vi "Test Message.vi"(8 "error in (no error)":errorcluster) -> (0 "error out":errorcluster)   [LabVIEW 2020]
uses:
  Source/Protobuf RAW/double/double.lvclass/double.ctl
  Source/Protobuf RAW/sint64/sint64.lvclass/sint64.ctl
  Source/Protobuf RAW/string/string.lvclass/string.ctl
  Source/Protobuf RAW/int32/int32.lvclass/int32.ctl
  Source/Protobuf RAW/sint64/Write Value.vi
  Source/Protobuf RAW/double/Write Value.vi
  Source/Protobuf RAW/string/Write Value.vi
  Source/Protobuf RAW/int32/Write Value.vi
  Source/Protobuf RAW/string/string.lvclass
  E:/Labview/LV 2020/Libs/LV Protobuf Raw/Source/Protobuf RAW/Tag/Basic Type.lvclass
  Source/Protobuf RAW/double/double.lvclass
  Source/Protobuf RAW/sint64/sint64.lvclass
  Source/Protobuf RAW/int32/int32.lvclass
  Source/Protobuf RAW/Message/New Raw Message.vi
  <vilib>/addons/_JKI Toolkits/Caraya/classes/Assert/Assert Equal Value_Variant.vi
  <vilib>/addons/_JKI Toolkits/Caraya/classes/Assert/Assert Not Equal Value_Variant.vi
  Source/Protobuf RAW/Message/Raw Message.lvclass
  Source/Protobuf RAW/Tag/Basic Type.lvclass
  <vilib>/addons/_JKI Toolkits/Caraya/classes/Test/Test.lvclass
  Source/Protobuf RAW.lvlib
  <vilib>/addons/_JKI Toolkits/Caraya/classes/Assert/Assert.lvclass
  E:/Labview/LV 2020/Libs/LV Protobuf Raw/Source/Protobuf RAW/Proto Value/Proto Type.lvclass
  E:/Labview/LV 2020/Libs/LV Protobuf Raw/Source/Protobuf RAW/Type Serializer/Type Serializer.lvclass
  E:/Labview/LV 2020/Libs/LV Protobuf Raw/Source/Protobuf RAW/String Representable/String Representable.lvclass
  E:/Labview/LV 2020/Libs/LV Protobuf Raw/Source/Protobuf RAW/Wire Type Group/Wire Type Group.lvclass
  E:/Labview/LV 2020/Libs/LV Protobuf Raw/Source/Protobuf RAW/LEN Encoder/LEN.lvclass
  E:/Labview/LV 2020/Libs/LV Protobuf Raw/Source/Protobuf RAW/string/string.lvclass
  E:/Labview/LV 2020/Libs/LV Protobuf Raw/Source/Protobuf RAW/Scalar Encoder/Scalar Type.lvclass
  E:/Labview/LV 2020/Libs/LV Protobuf Raw/Source/Protobuf RAW/VarINT Encoder/VarINT.lvclass
  E:/Labview/LV 2020/Libs/LV Protobuf Raw/Source/Protobuf RAW/int32/int32.lvclass
  E:/Labview/LV 2020/Libs/LV Protobuf Raw/Source/Protobuf RAW/I64 Wire/I64.lvclass
  E:/Labview/LV 2020/Libs/LV Protobuf Raw/Source/Protobuf RAW/double/double.lvclass
  E:/Labview/LV 2020/Libs/LV Protobuf Raw/Source/Protobuf RAW/Message/Raw Message.lvclass
  E:/Labview/LV 2020/Libs/LV Protobuf Raw/Source/Protobuf RAW/sint64/sint64.lvclass
panel:
  out "String Representation":string
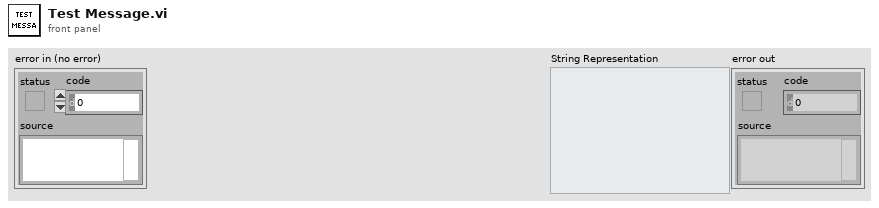
[diagram p1: front panel]
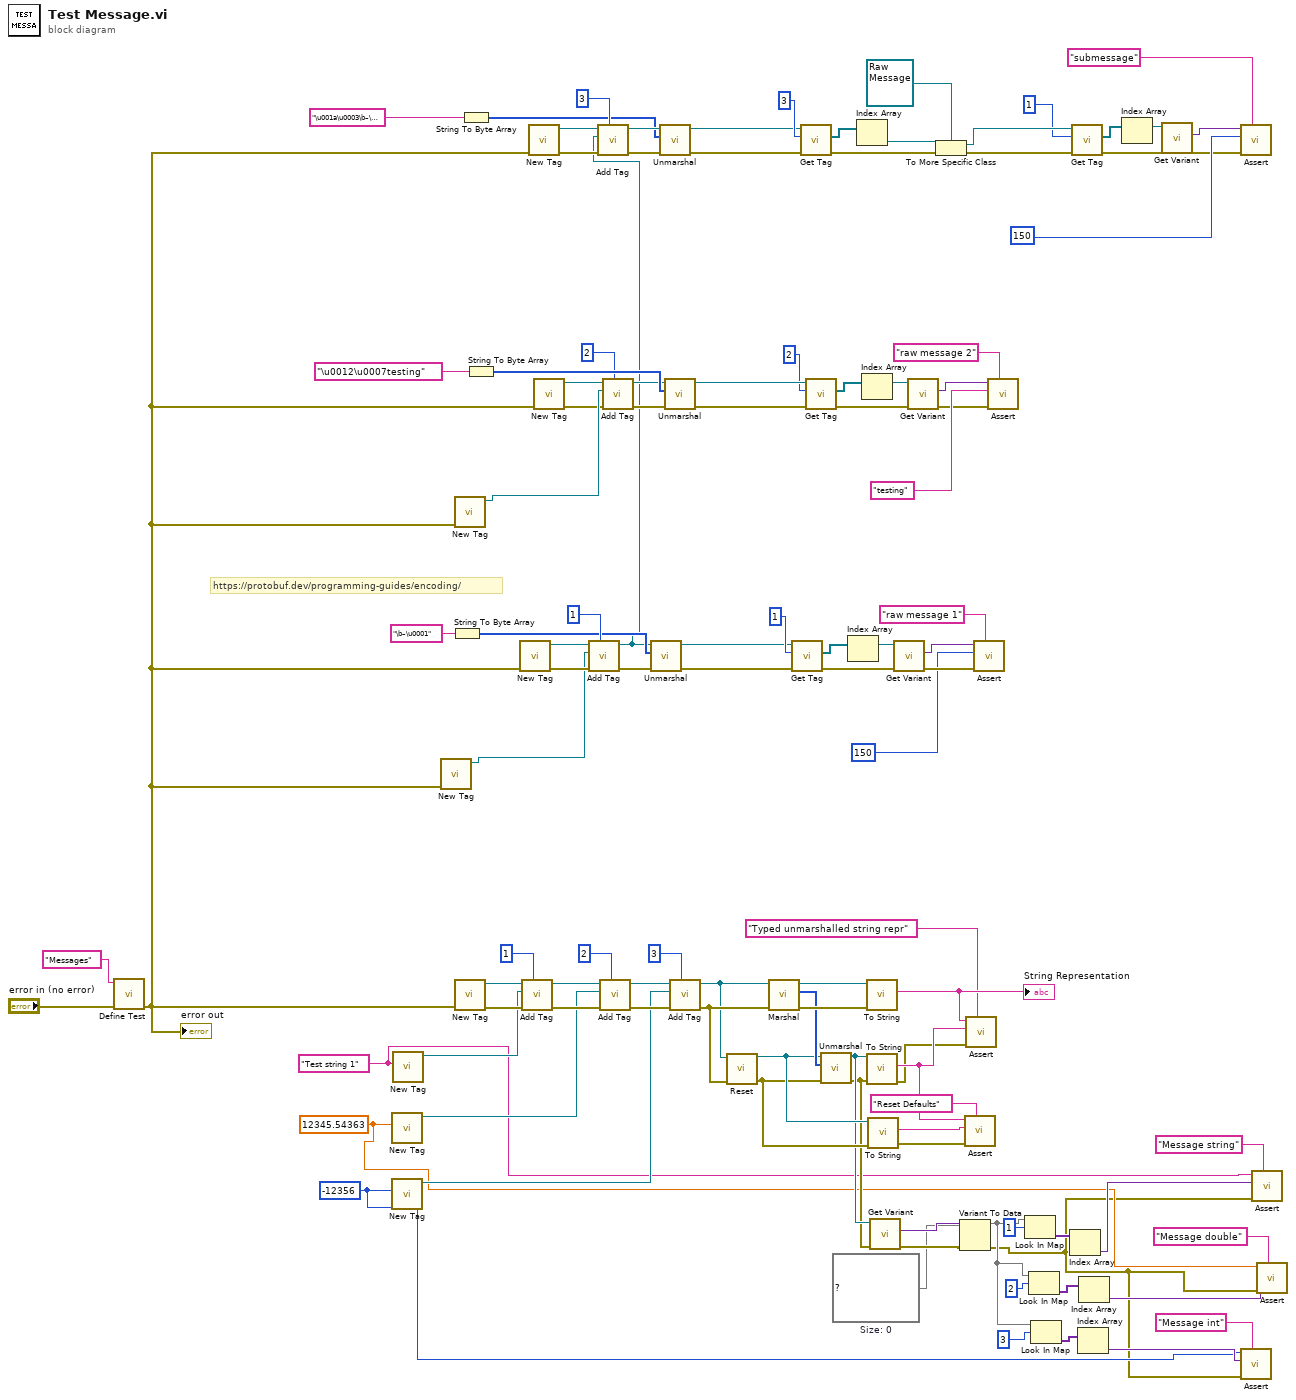
[diagram p0: block diagram]
diagram:
  w81 = map{u32, variant[]} {}  # Size: 0
  w69 = i64 -12356 ("Value")
  w68 = 12345.54363 ("Value")
  w73 = "Test string 1" ("Value")
  # "https://protobuf.dev/programming-guides/encoding/"
  n1 = call <vilib>:"Define Test.vi"("error in (no error)"="error in (no error)", "Label (VI Title)"="Messages") -> ("error out"=w12:errorcluster)  [unwired: 9 in]
  "error out" <- w12
  n2 = call-poly "New Tag.vi"("Value"=w68) -> ("double out"=w102:refnum<class "double.lvclass">)  [unwired: 9 in, 1 out]
  n3 = call-poly "New Tag.vi"("Value"=w69) -> ("int32 out"=w98:refnum<class "sint64.lvclass">)  [unwired: 9 in, 1 out]
  n4 = call-poly "New Tag.vi"("Value"=w73) -> ("string out"=w106:refnum<class "string.lvclass">)  [unwired: 9 in, 1 out]
  n5 = call-poly "New Tag.vi"("error in (no error)"=w12) -> ("int32 out"=w59:refnum<class "int32.lvclass">)  [unwired: 9 in, 1 out]
  n6 = String To Byte Array(string="\b–\u0001") -> (unsigned byte array=w48:u8[])
  n7 = call-poly "New Tag.vi"("error in (no error)"=w12) -> ("string out"=w30:refnum<class "string.lvclass">)  [unwired: 9 in, 1 out]
  n8 = call-poly "New Tag.vi"("error in (no error)"=w12) -> ("error out"=w108:errorcluster, "Raw Message out"=w109:refnum<class "Raw Message.lvclass">)  [unwired: 9 in]
  n9 = String To Byte Array(string="\u001a\u0003\b–\u0001") -> (unsigned byte array=w16:u8[])
  n10 = String To Byte Array(string="\u0012\u0007testing") -> (unsigned byte array=w41:u8[])
  n11 = call-poly "New Tag.vi"("error in (no error)"=w12) -> ("error out"=w60:errorcluster, "Raw Message out"=w61:refnum<class "Raw Message.lvclass">)  [unwired: 9 in]
  n12 = call-dynamic "Add Tag.vi"("ID"=u32 1, "error in (no error)"=w108, "Tag Value"=w106, "Message in"=w109) -> ("error out"=w105:errorcluster, "Message out"=w104:refnum<class "Raw Message.lvclass">)  [unwired: 6 in]
  n13 = call-poly "New Tag.vi"("error in (no error)"=w12) -> ("error out"=w24:errorcluster, "Raw Message out"=w25:refnum<class "Raw Message.lvclass">)  [unwired: 9 in]
  n14 = call-poly "New Tag.vi"("error in (no error)"=w12) -> ("error out"=w29:errorcluster, "Raw Message out"=w28:refnum<class "Raw Message.lvclass">)  [unwired: 9 in]
  n15 = call-dynamic "Add Tag.vi"("ID"=u32 1, "error in (no error)"=w60, "Tag Value"=w59, "Message in"=w61) -> ("error out"=w58:errorcluster, "Message out"=w13:refnum<class "Raw Message.lvclass">)  [unwired: 6 in]
  n16 = call-dynamic "Add Tag.vi"("ID"=u32 3, "error in (no error)"=w24, "Tag Value"=w13, "Message in"=w25) -> ("error out"=w23:errorcluster, "Message out"=w22:refnum<class "Raw Message.lvclass">)  [unwired: 6 in]
  n17 = call-dynamic "Add Tag.vi"("ID"=u32 2, "error in (no error)"=w105, "Tag Value"=w102, "Message in"=w104) -> ("error out"=w101:errorcluster, "Message out"=w100:refnum<class "Raw Message.lvclass">)  [unwired: 6 in]
  n18 = call-dynamic "Add Tag.vi"("ID"=u32 2, "error in (no error)"=w29, "Tag Value"=w30, "Message in"=w28) -> ("error out"=w31:errorcluster, "Message out"=w32:refnum<class "Raw Message.lvclass">)  [unwired: 6 in]
  n19 = call-dynamic "Unmarshal.vi"("error in (no error)"=w58, "Buffer"=w48, "Message in"=w13) -> ("error out"=w46:errorcluster, "Message out"=w47:refnum<class "Raw Message.lvclass">)  [unwired: 6 in, 1 out]
  n20 = call-dynamic "Unmarshal.vi"("error in (no error)"=w23, "Buffer"=w16, "Message in"=w22) -> ("error out"=w14:errorcluster, "Message out"=w15:refnum<class "Raw Message.lvclass">)  [unwired: 6 in, 1 out]
  n21 = call-dynamic "Unmarshal.vi"("error in (no error)"=w31, "Buffer"=w41, "Message in"=w32) -> ("error out"=w43:errorcluster, "Message out"=w42:refnum<class "Raw Message.lvclass">)  [unwired: 6 in, 1 out]
  n22 = call-dynamic "Add Tag.vi"("ID"=u32 3, "error in (no error)"=w101, "Tag Value"=w98, "Message in"=w100) -> ("error out"=w97:errorcluster, "Message out"=w91:refnum<class "Raw Message.lvclass">)  [unwired: 6 in]
  n23 = call-dynamic "Reset.vi"("error in (no error)"=w97, "Proto Tag in"=w91) -> ("error out"=w89:errorcluster, "Proto Tag out"=w90:refnum<class "Raw Message.lvclass">)  [unwired: 8 in]
  n24 = call-dynamic "Marshal.vi"("error in (no error)"=w97, "Message in"=w91) -> ("error out"=w95:errorcluster, "Buffer"=w94:u8[], "Message out"=w96:refnum<class "Raw Message.lvclass">)  [unwired: 7 in]
  n25 = call "Get Tag.vi"("error in (no error)"=w46, "ID"=u32 1, "Raw Message in"=w47) -> ("error out"=w57:errorcluster, "value"=w56:refnum<class "Basic Type.lvclass">[])  [unwired: 6 in, 1 out]
  n26 = call "Get Tag.vi"("error in (no error)"=w14, "ID"=u32 3, "Raw Message in"=w15) -> ("error out"=w21:errorcluster, "value"=w20:refnum<class "Basic Type.lvclass">[])  [unwired: 6 in, 1 out]
  n27 = call "Get Tag.vi"("error in (no error)"=w43, "ID"=u32 2, "Raw Message in"=w42) -> ("error out"=w33:errorcluster, "value"=w34:refnum<class "Basic Type.lvclass">[])  [unwired: 6 in, 1 out]
  n28 = call-dynamic "Unmarshal.vi"("error in (no error)"=w89, "Buffer"=w94, "Message in"=w90) -> ("error out"=w84:errorcluster, "Message out"=w85:refnum<class "Raw Message.lvclass">)  [unwired: 6 in, 1 out]
  n29 = Index Array(array=w56) -> (element=w55:refnum<class "Basic Type.lvclass">)  [unwired: 1 in]
  n30 = Index Array(array=w20) -> (element=w10:refnum<class "Basic Type.lvclass">)  [unwired: 1 in]
  n31 = Index Array(array=w34) -> (element=w35:refnum<class "Basic Type.lvclass">)  [unwired: 1 in]
  n32 = call-dynamic "To String.vi"("error in (no error)"=w95, "Raw Message in"=w96) -> ("String Representation"=w93:string)  [unwired: 7 in, 2 out]
  "String Representation" <- w93
  n33 = call-dynamic "To String.vi"("error in (no error)"=w84, "Raw Message in"=w85) -> ("error out"=w62:errorcluster, "String Representation"=w88:string)  [unwired: 7 in, 1 out]
  n34 = call-dynamic "To String.vi"("error in (no error)"=w89, "Raw Message in"=w90) -> ("error out"=w63:errorcluster, "String Representation"=w87:string)  [unwired: 7 in, 1 out]
  n35 = call-dynamic "Get Variant.vi"("error in (no error)"=w84, "Message in"=w85) -> ("error out"=w82:errorcluster, "Variant"=w83:variant)  [unwired: 7 in, 1 out]
  n36 = call-dynamic "Get Variant.vi"("error in (no error)"=w57, "Type Serializer in"=w55) -> ("error out"=w54:errorcluster, "Variant"=w53:variant)  [unwired: 7 in, 1 out]
  n37 = call-dynamic "Get Variant.vi"("error in (no error)"=w33, "Type Serializer in"=w35) -> ("error out"=w36:errorcluster, "Variant"=w37:variant)  [unwired: 7 in, 1 out]
  n38 = To More Specific Class(target class=refnum<class "Raw Message.lvclass"> refnum ("Message out"), reference=w10, error in=w21) -> (specific class reference=w9:refnum<class "Raw Message.lvclass">, error out=w11:errorcluster)
  n39 = Variant To Data(error in=w82, type=w81, Variant=w83) -> (data=w78:map{u32, variant[]}, error out=w64:errorcluster)
  n40 = call-poly <vilib>:"Assert.vi"("Label"="Reset Defaults", "error in (no error)"=w63, "Y"=w87, "X"=w88) -> ()  [unwired: 7 in, 1 out]
  n41 = call-poly <vilib>:"Assert.vi"("Label"="Typed unmarshalled string repr", "error in (no error)"=w62, "Y"=w88, "X"=w93) -> ()  [unwired: 7 in, 1 out]
  n42 = call-poly <vilib>:"Assert.vi"("Label"="raw message 1", "error in (no error)"=w54, "Y"=150 ("Value"), "X"=w53) -> ()  [unwired: 7 in, 1 out]
  n43 = call-poly <vilib>:"Assert.vi"("Label"="raw message 2", "error in (no error)"=w36, "Y"="testing" ("Value"), "X"=w37) -> ()  [unwired: 7 in, 1 out]
  n44 = Look In Map(map=w78, key=u32 1) -> (value=w76:variant[])  [unwired: 1 in, 1 out]
  n45 = Look In Map(map=w78, key=u32 2) -> (value=w75:variant[])  [unwired: 1 in, 1 out]
  n46 = Look In Map(map=w78, key=u32 3) -> (value=w74:variant[])  [unwired: 1 in, 1 out]
  n47 = Index Array(array=w76) -> (element=w72:variant)  [unwired: 1 in]
  n48 = call "Get Tag.vi"("error in (no error)"=w11, "ID"=u32 1, "Raw Message in"=w9) -> ("error out"=w5:errorcluster, "value"=w4:refnum<class "Basic Type.lvclass">[])  [unwired: 6 in, 1 out]
  n49 = Index Array(array=w74) -> (element=w70:variant)  [unwired: 1 in]
  n50 = Index Array(array=w75) -> (element=w71:variant)  [unwired: 1 in]
  n51 = Index Array(array=w4) -> (element=w3:refnum<class "Basic Type.lvclass">)  [unwired: 1 in]
  n52 = call-dynamic "Get Variant.vi"("error in (no error)"=w5, "Type Serializer in"=w3) -> ("error out"=w1:errorcluster, "Variant"=w2:variant)  [unwired: 7 in, 1 out]
  n53 = call-poly <vilib>:"Assert.vi"("Label"="submessage", "error in (no error)"=w1, "Y"=150 ("Value"), "X"=w2) -> ()  [unwired: 7 in, 1 out]
  n54 = call-poly <vilib>:"Assert.vi"("Label"="Message int", "error in (no error)"=w64, "Y"=w70, "X"=w69) -> ()  [unwired: 7 in, 1 out]
  n55 = call-poly <vilib>:"Assert.vi"("Label"="Message string", "error in (no error)"=w64, "Y"=w72, "X"=w73) -> ()  [unwired: 7 in, 1 out]
  n56 = call-poly <vilib>:"Assert.vi"("Label"="Message double", "error in (no error)"=w64, "Y"=w71, "X"=w68) -> ()  [unwired: 7 in, 1 out]
